vi "氨氮通讯.vi"() -> ()   [LabVIEW 2016, in "斯坦道氨氮.lvlib"]
uses:
  <vilib>/Plasmionique/MB Master/MB_Master_TCP/MB_Master_TCP.lvclass
  D:/Program Files (x86)/National Instruments/LabVIEW 2016/vi.lib/Plasmionique/MB Master/MB_Master/MB_Master.lvclass
  <vilib>/Utility/config.llb/Write Key (String).vi
  <vilib>/Plasmionique/MB Master/MB_Master/MB_Master.lvclass
  <vilib>/Utility/config.llb/NI_LVConfig.lvlib
  <vilib>/Plasmionique/MB Master/MB Master.lvlib
panel:
  out "序列号":string
  out "状态告警区":T1
  out "status":bool
  out "关键参数区":T2
  in  "读关键参数区":bool
  in  "读状态告警区":bool
  in  "读测量数据区":bool
  in  "站号":u16(ring) items=["总磷"=1, "氨氮"=3]
  in  "停止":bool
  in  "启动":bool
  in  "控制命令":u16(ring) items=["启动测量"=1, "标样核查"=2, "零点核查"=3, "跨度核查"=4, "空白测试"=5, "平行样测试"=6, "加标回收"=7, "空白校准"=8, "标样校准"=9, "初始化（清洗）"=10, "停止测试"=11, "仪器重启"=12, "校时"=13, "模式设置"=14, "测量间隔设置"=15]
  in  "控制命令参数":u16[](array[numeric]) format="%04xH"
  in  "VISA Resource":refnum<visa-resource-name>
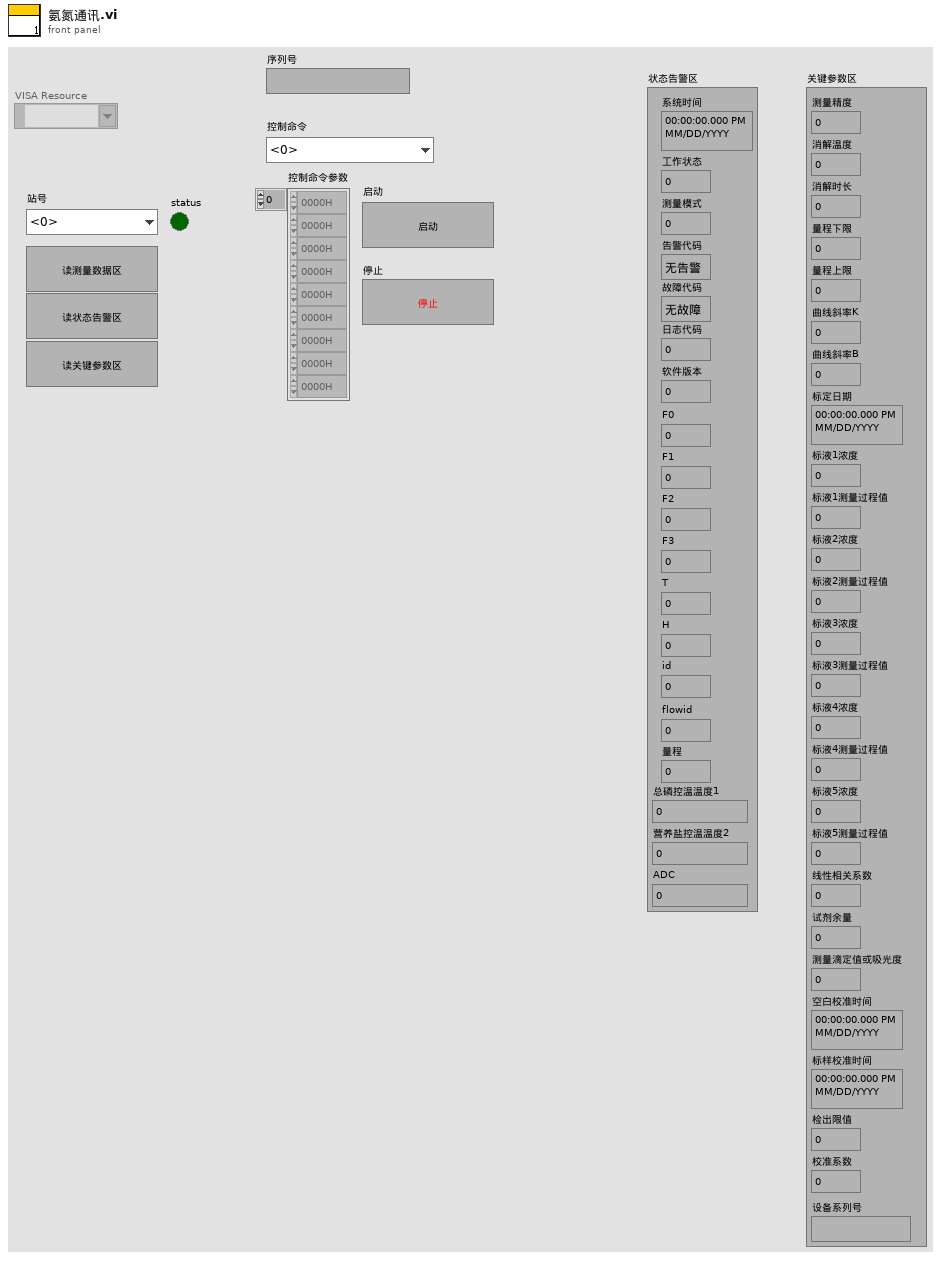
[diagram p1: front panel]
types:
  T1 = cluster{"系统时间":timestamp, "工作状态":u16, "测量模式":u16, "告警代码":enum16{"无告警", "缺试剂告警", "缺水样告警", "缺蒸馏水告警", "缺标液告警", "仪表漏液告警", "标定异常告警", "超量程告警", "加热异常", "低试剂预警", "超上限告警", "超下限告警", "仪表内部其他异常", "滴定异常告警", "电极异常告警", "量程切换告警", "参数设置告警", "PH电极电位异常", "电导率电极异常", "浊度光度异常", "溶解氧电极异常", "溶解氧光强异常", "温度异常告警", "PH异常告警", "溶解氧异常告警", "电导率异常告警", "浊度异常告警", "叶绿素异常告警", "藻密度异常告警", "蓝绿藻异常告警", "ORP异常告警", "氨氮异常告警", "清洁刷异常告警", "SD卡异常告警", "蓝牙异常告警", "Wifi异常告警", "流程异常告警"}, "故障代码":enum16{"无故障", "电机故障", "温度故障", "通讯故障", "滴定故障"}, "日志代码":u16, "软件版本":u16, "F0":sgl, "F1":sgl, "F2":sgl, "F3":sgl, "T":sgl, "H":sgl, "id":u16, "flowid":u16, "量程":u16, "ADC":sgl, "营养盐控温温度2":sgl, "总磷控温温度1":sgl}
  T2 = cluster{"测量精度":u16, "消解温度":u16, "消解时长":u16, "量程下限":sgl, "量程上限":sgl, "曲线斜率K":sgl, "曲线斜率B":sgl, "标定日期":timestamp, "标液1浓度":sgl, "标液1测量过程值":sgl, "标液2浓度":sgl, "标液2测量过程值":sgl, "标液3浓度":sgl, "标液3测量过程值":sgl, "标液4浓度":sgl, "标液4测量过程值":sgl, "标液5浓度":sgl, "标液5测量过程值":sgl, "线性相关系数":sgl, "试剂余量":u32, "测量滴定值或吸光度":sgl, "空白校准时间":timestamp, "标样校准时间":timestamp, "检出限值":sgl, "校准系数":sgl, "设备系列号":string}
  T3 = typedef "NI_LVConfig.lvlib/Config Data RefNum.ctl" = refnum<k1>
  T4 = enum8{"Enabled", "Disabled", "Disabled and Grayed Out"}
  T5 = cluster{"因子编码":u32, "单位":u16, "标样参考值":sgl, "水样数据时间":timestamp, "水样实测值":sgl, "水样数据标识":string, "标样数据时间":timestamp, "标样实测值":sgl, "标样数据标识":string, "空白数据时间":timestamp, "空白实测值":sgl, "空白数据标识":string, "零点核查数据时间":timestamp, "零点核查实测值":sgl, "零点核查数据标识":string, "跨度核查数据时间":timestamp, "跨度核查实测值":sgl, "跨度核查数据标识":string, "加标回收数据时间":timestamp, "加标回收实测值":sgl, "加标回收数据标识":string, "平行样数据时间":timestamp, "平行样实测值":sgl, "平行样数据标识":string, "F0":sgl, "F1":sgl, "F2":sgl, "F3":sgl, "F4":sgl, "F5":sgl, "F6":sgl, "F7":sgl, "温度":sgl, "湿度":sgl, "X值":sgl}
  T6 = cluster{"系统时间":timestamp, "工作状态":enum16{"空闲", "水样测试", "标样核查", "零点核查", "跨度核查", "空白测试", "平行样测试", "加标回收", "空白校准", "标样校准", "初始化（清洗）"}, "测量模式":enum16{"待机", "连续模式", "周期模式", "定点模式", "受控模式", "手动模式"}, "告警代码":enum16{"无告警", "缺试剂告警", "缺水样告警", "缺蒸馏水告警", "缺标液告警", "仪表漏液告警", "标定异常告警", "超量程告警", "加热异常", "低试剂预警", "超上限告警", "超下限告警", "仪表内部其他异常", "滴定异常告警", "电极异常告警", "量程切换告警", "参数设置告警", "PH电极电位异常", "电导率电极异常", "浊度光度异常", "溶解氧电极异常", "溶解氧光强异常", "温度异常告警", "PH异常告警", "溶解氧异常告警", "电导率异常告警", "浊度异常告警", "叶绿素异常告警", "藻密度异常告警", "蓝绿藻异常告警", "ORP异常告警", "氨氮异常告警", "清洁刷异常告警", "SD卡异常告警", "蓝牙异常告警", "Wifi异常告警", "流程异常告警"}, "故障代码":enum16{"无故障", "电机故障", "温度故障", "通讯故障", "滴定故障"}, "日志代码":u16, "软件版本":u16, "F0":sgl, "F1":sgl, "F2":sgl, "F3":sgl, "T":sgl, "H":sgl, "id":u16, "flowid":u16, "量程":u16, "总磷控温温度1":sgl, "营养盐控温温度2":sgl, "ADC":sgl}
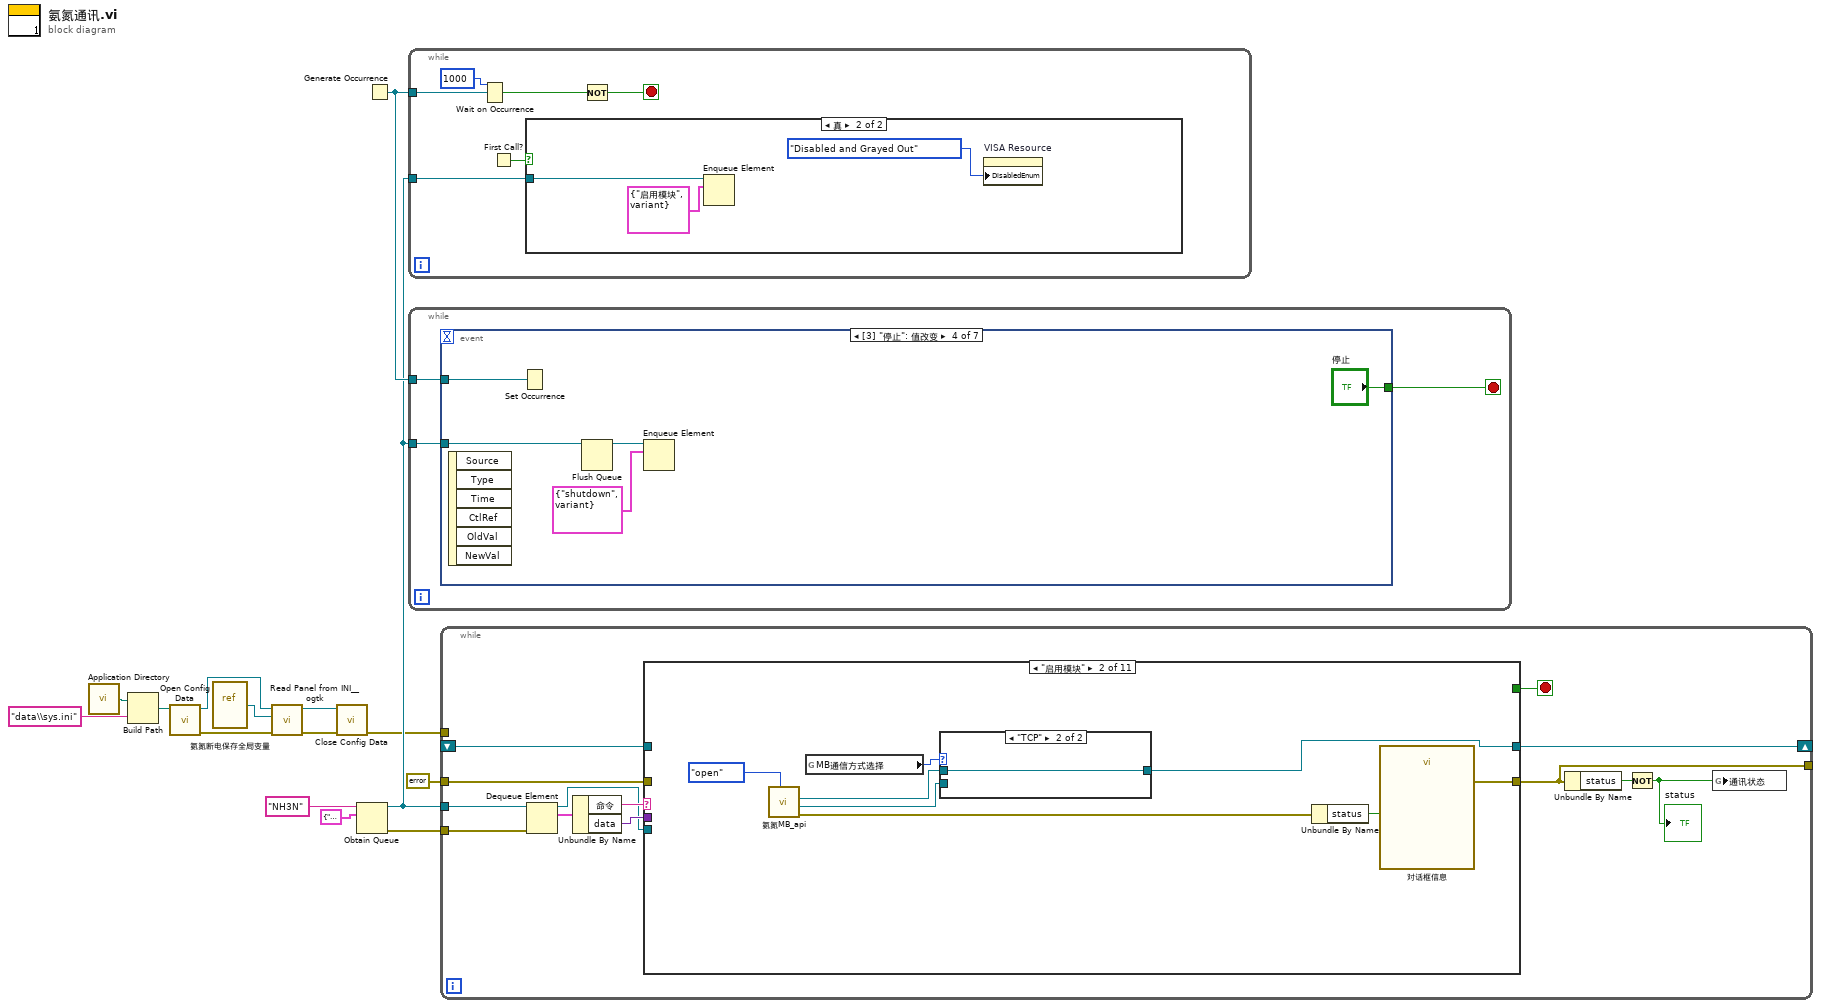
[diagram p0: block diagram]
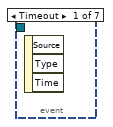
[diagram p3: hidden frame]
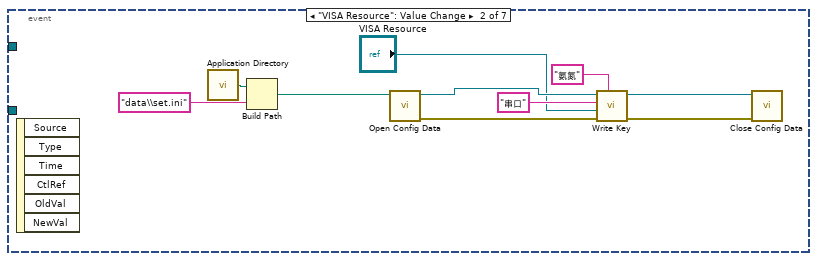
[diagram p4: hidden frame]
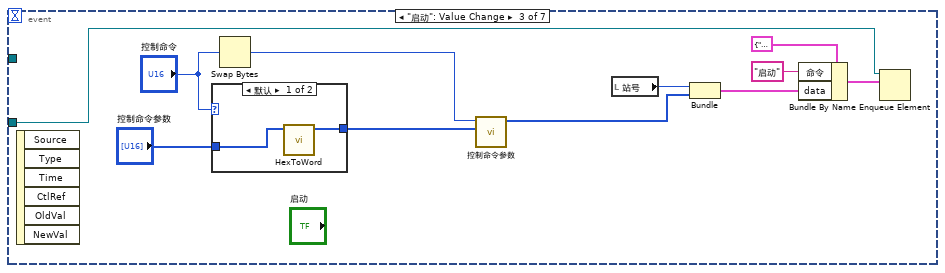
[diagram p5: hidden frame]
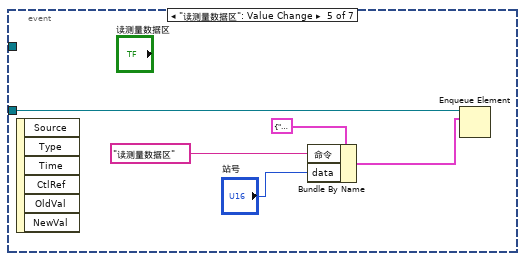
[diagram p7: hidden frame]
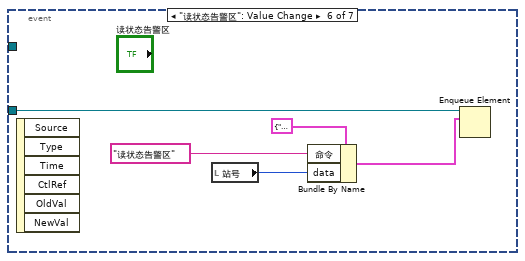
[diagram p8: hidden frame]
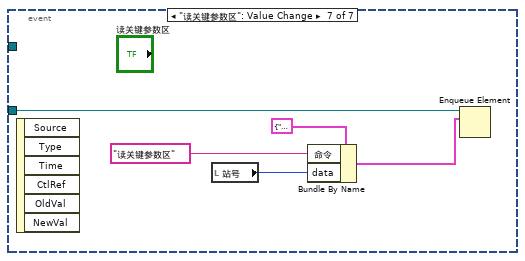
[diagram p9: hidden frame]
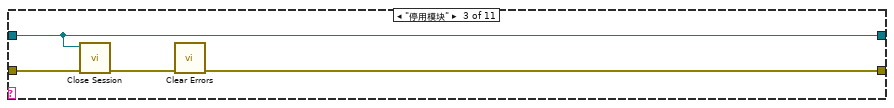
[diagram p12: hidden frame]
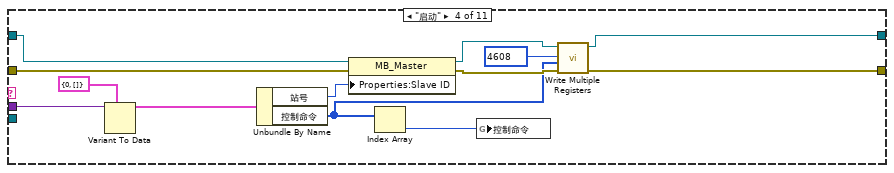
[diagram p13: hidden frame]
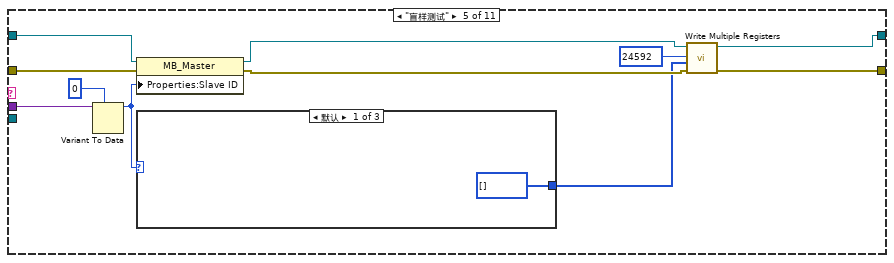
[diagram p14: hidden frame]
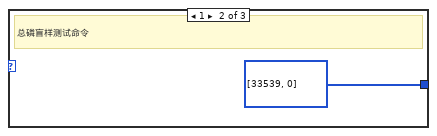
[diagram p15: hidden frame]
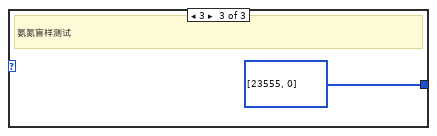
[diagram p16: hidden frame]
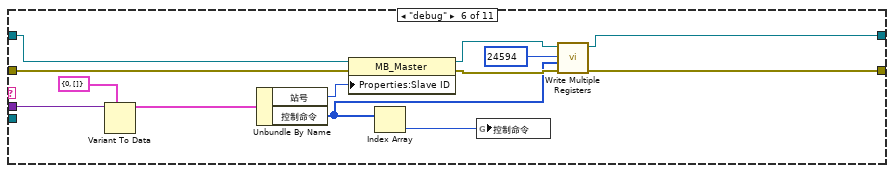
[diagram p17: hidden frame]
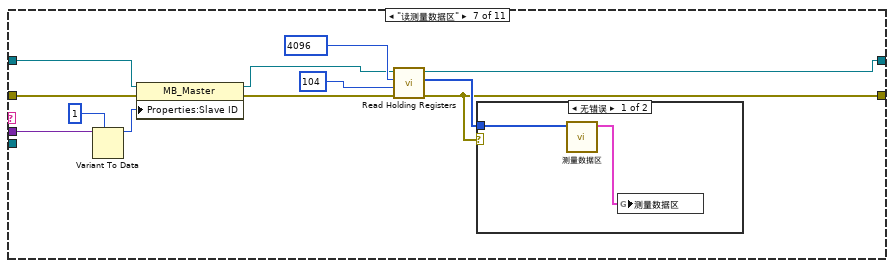
[diagram p18: hidden frame]
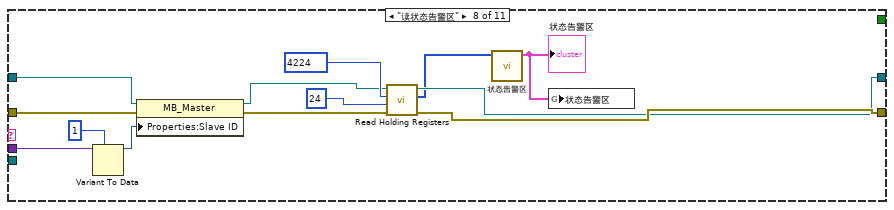
[diagram p20: hidden frame]
diagram:
  n1 = call <vilib>:"Application Directory.vi"() -> ("Application Directory"=w2:path)
  n2 = Build Path(base path=w2, name or relative path="data\\sys.ini" ("名称或相对路径")) -> (appended path=w4:path)
  n3 = call <vilib>:"Open Config Data.vi"("configuration file path"=w4) -> ("error out"=w8:errorcluster, "refnum"=w5:T3)  [unwired: 8 in, 1 out]
  n4 = vi-ref "氨氮断电保存全局变量.vi"() -> (w6:refnum<vi>)
  n5 = call <userlib>:"Read Panel from INI__ogtk.vi"("error in (no error)"=w8, "VI ref"=w6, "refnum"=w5) -> ("error out"=w9:errorcluster, "refnum out"=w7:T3)  [unwired: 7 in]
  n6 = call <vilib>:"Close Config Data.vi"("error in (no error)"=w9, "refnum"=w7) -> ("error out"=w1:errorcluster)  [unwired: 8 in, 1 out]
  n7 = Obtain Queue(name (unnamed)="NH3N" ("名称（未命名）"), element data type=cluster{"命令":string, "data":variant} {"命令"="", "data"=variant}) -> (queue out=w10:refnum<queue>, error out=w13:errorcluster)  [unwired: 3 in, 1 out]
  n8 = Generate Occurrence() -> (w11:refnum<k4>)
  n9 = while {
    tunnel: w11 -> [w21]
    tunnel: w10 -> [w17]
    stop <- w18 stop-if-true
    n10 = Wait on Occurrence(2:w21, 3:1000 ("毫秒超时(-1)")) -> (0:w19:bool)  [unwired: 1 in]
    n11 = First Call?() -> (First Call?: T/F=w16:bool)
    n12 = case shown="真" w16 {
      tunnel: w17 -> [_ w23]
      frame False {
      }
      frame True {
        n13 = Enqueue Element(queue=w23, element=cluster{"命令":string, "data":variant} {"命令"="启用模块", "data"=variant} ("元素")) -> ()  [unwired: 2 in, 3 out]
        n14 = property on="VISA Resource" class="VISAName"("DisabledEnum"=T4."Disabled and Grayed Out" ("禁用")) -> ()  [unwired: 2 in, 2 out]
      }
    }
    n15 = Not(x=w19) -> (.not. x?=w18:bool)
  }
  n16 = while {
    tunnel: w10 -> [w27]
    tunnel: w11 -> [w25]
    stop <- w26 stop-if-true
    n17 = event shown="[3] \"停止\": 值改变" {
      selector: _ -> [_ _ _ _ _ _ _]
      dyn-events: _ -> [_ _ _ _ _ _ _]
      timeout: _ -> [_ _ _ _ _ _ _]
      tunnel: w27 -> [_ _ w48 w55 w61 w66 w71]
      tunnel: [_ _ _ "停止" _ _ _] -> w26
      tunnel: w25 -> [_ _ _ w52 _ _ _]
      event Timeout {
        n18 = event-data() -> ()  [unwired: 1 in, 3 out]
      }
      event "VISA Resource": Value Change {
        n19 = event-data() -> ()  [unwired: 1 in, 6 out]
        n20 = call <vilib>:"Application Directory.vi"() -> ("Application Directory"=w30:path)
        n21 = Build Path(base path=w30, name or relative path="data\\set.ini" ("名称或相对路径")) -> (appended path=w31:path)
        n22 = call <vilib>:"Open Config Data.vi"("configuration file path"=w31) -> ("error out"=w37:errorcluster, "refnum"=w36:T3)  [unwired: 8 in, 1 out]
        n23 = call-poly <vilib>:"Write Key.vi"("section"="氨氮", "error in (no error)"=w37, "value"="VISA Resource", "key"="串口", "refnum"=w36) -> ("error out"=w33:errorcluster, "refnum out"=w29:T3)  [unwired: 4 in, 1 out]
        n24 = call <vilib>:"Close Config Data.vi"("error in (no error)"=w33, "refnum"=w29) -> ()  [unwired: 8 in, 2 out]
      }
      event "启动": Value Change {
        n25 = event-data() -> ()  [unwired: 1 in, 6 out]
        n26 = case shown="默认" "控制命令" {
          tunnel: "控制命令参数" -> [w50 w51]
          tunnel: [w49 w51] -> w38
          frame Default {
            n27 = call "HexToWord.vi"("数组"=w50) -> ("WORD"=w49:u16[])  [unwired: 10 in]
          }
          frame 13 {
          }
        }
        n28 = Swap Bytes(anything="控制命令") -> (byte swapped=w41:u16)
        n29 = call "控制命令参数.vi"("控制命令参数"=w38, "控制命令"=w41) -> ("控制命令输出"=w44:u16[])  [unwired: 9 in]
        n30 = local read "站号"() -> (w43:u16)
        n31 = Bundle("站号"=w43, "控制命令输出"=w44) -> (w42:cluster{"站号":u16, "控制命令输出":u16[]})  [unwired: 1 in]
        n32 = Bundle By Name(cluster=cluster{"命令":string, "data":variant} {"命令"="", "data"=variant} ("元素"), "命令"="启动", "data"=w42) -> (w46:cluster{"命令":string, "data":variant})
        n33 = Enqueue Element(queue=w48, element=w46) -> ()  [unwired: 2 in, 3 out]
      }
      event "停止": Value Change {
        n34 = event-data() -> ()  [unwired: 1 in, 6 out]
        n35 = Set Occurrence(w52) -> ()
        n36 = Flush Queue(queue=w55) -> (queue out=w54:refnum<queue>)  [unwired: 1 in, 2 out]
        n37 = Enqueue Element(queue=w54, element=cluster{"命令":string, "data":variant} {"命令"="shutdown", "data"=variant} ("元素")) -> ()  [unwired: 2 in, 3 out]
      }
      event "读测量数据区": Value Change {
        n38 = event-data() -> ()  [unwired: 1 in, 6 out]
        n39 = Bundle By Name(cluster=cluster{"命令":string, "data":variant} {"命令"="", "data"=variant} ("元素"), "命令"="读测量数据区", "data"="站号") -> (w59:cluster{"命令":string, "data":variant})
        n40 = Enqueue Element(queue=w61, element=w59) -> ()  [unwired: 2 in, 3 out]
      }
      event "读状态告警区": Value Change {
        n41 = event-data() -> ()  [unwired: 1 in, 6 out]
        n42 = local read "站号"() -> (w62:u16)
        n43 = Bundle By Name(cluster=cluster{"命令":string, "data":variant} {"命令"="", "data"=variant} ("元素"), "命令"="读状态告警区", "data"=w62) -> (w64:cluster{"命令":string, "data":variant})
        n44 = Enqueue Element(queue=w66, element=w64) -> ()  [unwired: 2 in, 3 out]
      }
      event "读关键参数区": Value Change {
        n45 = event-data() -> ()  [unwired: 1 in, 6 out]
        n46 = local read "站号"() -> (w67:u16)
        n47 = Bundle By Name(cluster=cluster{"命令":string, "data":variant} {"命令"="", "data"=variant} ("元素"), "命令"="读关键参数区", "data"=w67) -> (w69:cluster{"命令":string, "data":variant})
        n48 = Enqueue Element(queue=w71, element=w69) -> ()  [unwired: 2 in, 3 out]
      }
    }
  }
  n49 = while {
    tunnel: w10 -> [w84]
    tunnel: w13 -> [w83]
    shift-right: [w81] -> _
    shift-left: _ -> [w80]
    tunnel: errorcluster {"status"=FALSE, "code"=0, "source"=""} ("error out") -> [w79]
    tunnel: [w74] -> _
    tunnel: w1 -> [_]
    stop <- w82 stop-if-true
    n50 = Dequeue Element(queue=w84, error in (no error)=w83) -> (queue out=w75:refnum<queue>, element=w77:cluster{"命令":string, "data":variant})  [unwired: 1 in, 2 out]
    n51 = Unbundle By Name(w77) -> ("命令"=w78:string, "data"=w76:variant)
    n52 = case shown="\"启用模块\"" w78 {
      tunnel: w76 -> [_ _ _ w110 w121 w138 w147 w157 w172 w186 _]
      tunnel: w75 -> [_ _ _ _ _ _ _ _ _ _ w199]
      tunnel: [_ _ _ _ _ _ _ _ _ _ TRUE] -> w82
      tunnel: [w85 w87 w97 w113 w124 w140 w152 w166 w179 w193 w195] -> w81
      tunnel: [w86 w93 w98 w112 w123 w139 w141 w167 w180 w194 w196] -> w74
      tunnel: w80 -> [w85 _ w97 w109 w120 w137 w146 w160 w175 w189 w195]
      tunnel: w79 -> [w86 _ w100 w106 w117 w134 w144 w161 w176 w190 w197]
      frame Default {
      }
      frame "启用模块" {
        n53 = call "氨氮MB_api.vi"("STEP"=enum16{"open", "read", "write", "close"}."open") -> ("error out"=w91:errorcluster, "MB session out"=w88:refnum<class "MB_Master.lvclass">, "MB_TCP session"=w89:refnum<class "MB_Master_TCP.lvclass">)  [unwired: 7 in, 1 out]
        n54 = global read "氨氮断电保存全局变量.vi" "MB通信方式选择"() -> (w90:enum16{"串口", "TCP"})
        n55 = case shown="\"TCP\"" w90 {
          tunnel: w89 -> [_ w96]
          tunnel: w88 -> [w95 _]
          tunnel: [w95 w96] -> w87
          frame "串口", Default {
          }
          frame "TCP" {
          }
        }
        n56 = Unbundle By Name(w91) -> ("status"=w94:bool)
        n57 = call "对话框信息"("Enable"=w94) -> ("error out"=w93:errorcluster)  [unwired: 9 in, 1 out]
      }
      frame "停用模块" {
        n58 = call-dynamic "Close Session.vi"("error in (no error)"=w100, "MB session in"=w97) -> ("error out"=w99:errorcluster)  [unwired: 9 in]
        n59 = call <vilib>:"Clear Errors.vi"("error in (no error)"=w99) -> ("error out"=w98:errorcluster)  [unwired: 5 in, 1 out]
      }
      frame "启动" {
        n60 = Variant To Data(type=cluster{"站号":u16, "控制命令":u16[]} {"站号"=0, "控制命令"=[]} ("输出簇"), Variant=w110) -> (data=w104:cluster{"站号":u16, "控制命令":u16[]})  [unwired: 1 in, 1 out]
        n61 = Unbundle By Name(w104) -> ("站号"=w103:u16, "控制命令"=w101:u16[])
        n62 = property class="MB_Master"(reference=w109, error in=w106, "Properties:Slave ID"=w103) -> (reference out=w108:refnum<class "MB_Master.lvclass">, error out=w107:errorcluster)
        n63 = Index Array(array=w101) -> (element=w102:u16)  [unwired: 1 in]
        n64 = global write "VAR氨氮全局变量.vi" "控制命令"(w102) -> ()
        n65 = call <vilib>:"Write Multiple Registers.vi"("error in (no error)"=w107, "values"=w101, "starting address"=u16 4608, "MB session in"=w108) -> ("error out"=w112:errorcluster, "MB session out"=w113:refnum<class "MB_Master.lvclass">)  [unwired: 6 in]
      }
      frame "盲样测试" {
        n66 = Variant To Data(type=0, Variant=w121) -> (data=w114:i32)  [unwired: 1 in, 1 out]
        n67 = property class="MB_Master"(reference=w120, error in=w117, "Properties:Slave ID"=w114) -> (reference out=w119:refnum<class "MB_Master.lvclass">, error out=w118:errorcluster)
        n68 = case shown="默认" w114 {
          tunnel: [u16[] [] ("values") u16[] [33539, 0] ("values") u16[] [23555, 0] ("values")] -> w116
          frame Default {
          }
          frame 1 {
            # "总磷盲样测试命令"
          }
          frame 3 {
            # "氨氮盲样测试"
          }
        }
        n69 = call <vilib>:"Write Multiple Registers.vi"("error in (no error)"=w118, "values"=w116, "starting address"=u16 24592, "MB session in"=w119) -> ("error out"=w123:errorcluster, "MB session out"=w124:refnum<class "MB_Master.lvclass">)  [unwired: 6 in]
      }
      frame "debug" {
        n70 = Variant To Data(type=cluster{"站号":u16, "控制命令":u16[]} {"站号"=0, "控制命令"=[]} ("输出簇"), Variant=w138) -> (data=w132:cluster{"站号":u16, "控制命令":u16[]})  [unwired: 1 in, 1 out]
        n71 = Unbundle By Name(w132) -> ("站号"=w131:u16, "控制命令"=w129:u16[])
        n72 = property class="MB_Master"(reference=w137, error in=w134, "Properties:Slave ID"=w131) -> (reference out=w136:refnum<class "MB_Master.lvclass">, error out=w135:errorcluster)
        n73 = Index Array(array=w129) -> (element=w130:u16)  [unwired: 1 in]
        n74 = global write "VAR氨氮全局变量.vi" "控制命令"(w130) -> ()
        n75 = call <vilib>:"Write Multiple Registers.vi"("error in (no error)"=w135, "values"=w129, "starting address"=u16 24594, "MB session in"=w136) -> ("error out"=w139:errorcluster, "MB session out"=w140:refnum<class "MB_Master.lvclass">)  [unwired: 6 in]
      }
      frame "读测量数据区" {
        n76 = Variant To Data(type=u8 1 ("Slave ID"), Variant=w147) -> (data=w148:u8)  [unwired: 1 in, 1 out]
        n77 = property class="MB_Master"(reference=w146, error in=w144, "Properties:Slave ID"=w148) -> (reference out=w145:refnum<class "MB_Master.lvclass">, error out=w143:errorcluster)
        n78 = call <vilib>:"Read Holding Registers.vi"("error in (no error)"=w143, "quantity"=u16 104, "starting address"=u16 4096, "MB session in"=w145) -> ("error out"=w141:errorcluster, "Registers"=w142:u16[], "MB session out"=w152:refnum<class "MB_Master.lvclass">)  [unwired: 5 in]
        n79 = case shown="无错误" w141 {
          tunnel: w142 -> [w154 _]
          frame No Error {
            n80 = call "测量数据区.vi"("数组"=w154) -> ("测量数据区"=w153:T5)  [unwired: 10 in]
            n81 = global write "VAR氨氮全局变量.vi" "测量数据区"(w153) -> ()
          }
          frame Error {
          }
        }
      }
      frame "读状态告警区" {
        n82 = Variant To Data(type=u8 1 ("Slave ID"), Variant=w157) -> (data=w162:u8)  [unwired: 1 in, 1 out]
        n83 = property class="MB_Master"(reference=w160, error in=w161, "Properties:Slave ID"=w162) -> (reference out=w159:refnum<class "MB_Master.lvclass">, error out=w158:errorcluster)
        n84 = call <vilib>:"Read Holding Registers.vi"("error in (no error)"=w158, "quantity"=u16 24, "starting address"=u16 4224, "MB session in"=w159) -> ("error out"=w167:errorcluster, "Registers"=w156:u16[], "MB session out"=w166:refnum<class "MB_Master.lvclass">)  [unwired: 5 in]
        n85 = call "状态告警区.vi"("数组"=w156) -> ("状态告警区"=w155:T6)  [unwired: 10 in]
        "状态告警区" <- w155
        n86 = global write "VAR氨氮全局变量.vi" "状态告警区"(w155) -> ()
      }
      frame "读关键参数区" {
        n87 = Variant To Data(type=u8 1 ("Slave ID"), Variant=w172) -> (data=w170:u8)  [unwired: 1 in, 1 out]
        n88 = property class="MB_Master"(reference=w175, error in=w176, "Properties:Slave ID"=w170) -> (reference out=w174:refnum<class "MB_Master.lvclass">, error out=w173:errorcluster)
        n89 = call <vilib>:"Read Holding Registers.vi"("error in (no error)"=w173, "quantity"=u16 19, "starting address"=u16 4256, "MB session in"=w174) -> ("error out"=w180:errorcluster, "Registers"=w169:u16[], "MB session out"=w179:refnum<class "MB_Master.lvclass">)  [unwired: 5 in]
        n90 = call "关键参数区.vi"("数组"=w169) -> ("关键参数区"=w168:T2)  [unwired: 10 in]
        "关键参数区" <- w168
        n91 = global write "VAR氨氮全局变量.vi" "关键参数区"(w168) -> ()
      }
      frame "读序列号" {
        n92 = Variant To Data(type=u8 1 ("Slave ID"), Variant=w186) -> (data=w184:u8)  [unwired: 1 in, 1 out]
        n93 = property class="MB_Master"(reference=w189, error in=w190, "Properties:Slave ID"=w184) -> (reference out=w188:refnum<class "MB_Master.lvclass">, error out=w187:errorcluster)
        n94 = call <vilib>:"Read Holding Registers.vi"("error in (no error)"=w187, "quantity"=u16 6, "starting address"=u16 3, "MB session in"=w188) -> ("error out"=w194:errorcluster, "Registers"=w183:u16[], "MB session out"=w193:refnum<class "MB_Master.lvclass">)  [unwired: 5 in]
        n95 = call "HexToString.vi"("数组"=w183) -> ("STRING"=w182:string[])  [unwired: 10 in]
        n96 = Index Array(array=w182) -> (element=w181:string)  [unwired: 1 in]
        "序列号" <- w181
        n97 = global write "VAR氨氮全局变量.vi" "序列号"(w181) -> ()
      }
      frame "shutdown" {
        n98 = call-dynamic "Close Session.vi"("error in (no error)"=w197, "MB session in"=w195) -> ("error out"=w196:errorcluster)  [unwired: 9 in]
        n99 = Flush Queue(queue=w199) -> (queue out=w198:refnum<queue>)  [unwired: 1 in, 2 out]
        n100 = Release Queue(queue=w198) -> ()  [unwired: 2 in, 3 out]
      }
    }
    n101 = Unbundle By Name(w74) -> ("status"=w73:bool)
    n102 = Not(x=w73) -> (.not. x?=w72:bool)
    "status" <- w72
    n103 = global write "VAR氨氮全局变量.vi" "通讯状态"(w72) -> ()
  }
